vi "To String.vi"(8 "error in (no error)":errorcluster, 11 "String in":refnum<class "Path.lvclass">) -> (0 "error out":errorcluster, 2 "String":string)   [LabVIEW 2020, in "Data.lvlib" / "Path.lvclass"]
doc: "Convert 'Generic Data in' to a string.\nThe default implementation convert the data to an XML string."
uses:
  Path.lvclass
  Path.lvclass/Path.ctl
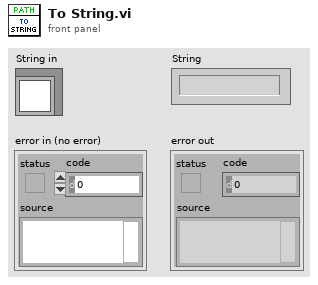
[diagram p1: front panel]
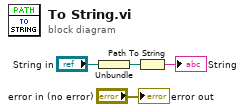
[diagram p0: block diagram]
diagram:
  n1 = Unbundle("String in") -> (w2:path)
  n2 = Path To String(path=w2) -> (string=→"String":string)
  "error out" <- "error in (no error)"
